vi "PreProcess.vi"(8 "error in (no error)":errorcluster, 11 "Input":T2) -> (0 "error out":errorcluster, 3 "Output":T1)   [LabVIEW 2023]
uses:
  <userlib>/WebService/_PreProcess/PreProcess.lvlib
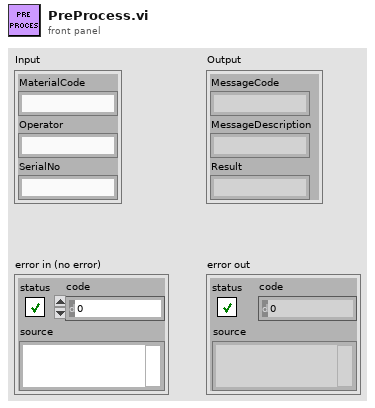
[diagram p1: front panel]
types:
  T1 = cluster{"MessageCode":string, "MessageDescription":string, "Result":string}
  T2 = cluster{"MaterialCode":string, "Operator":string, "SerialNo":string}
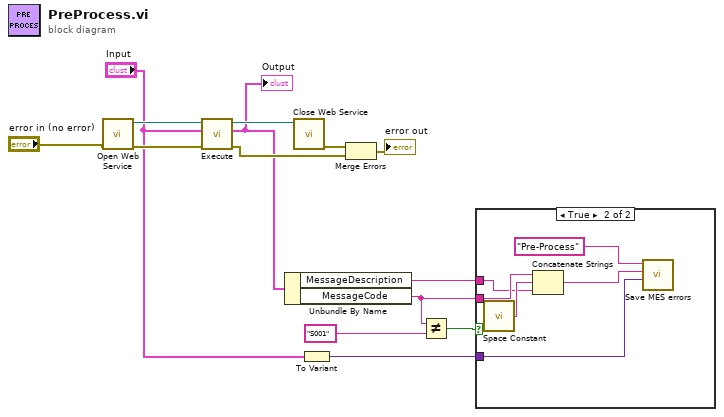
[diagram p0: block diagram]
diagram:
  n1 = call <userlib>:"Open Web Service.vi"("error in (no error)"="error in (no error)") -> ("error out"=w13:errorcluster, "PreProcess refnum"=w14:refnum<k24>)  [unwired: 9 in]
  n2 = call <userlib>:"Execute.vi"("error in (no error)"=w13, ".NET:CheckPqmNtrsAndProductSerialDateService.PqmNtrsAndProductSerialRequest"="Input", "PreProcess refnum"=w14) -> ("error out"=w8:errorcluster, ".NET:CheckPqmNtrsAndProductSerialDateService.CommonResponse"=w2:T1, "PreProcess refnum out"=w12:refnum<k24>)  [unwired: 6 in]
  "Output" <- w2
  n3 = Unbundle By Name(w2) -> ("MessageDescription"=w5:string, "MessageCode"=w4:string)
  n4 = call <userlib>:"Close Web Service.vi"("PreProcess refnum"=w12) -> ("error out"=w10:errorcluster)  [unwired: 10 in]
  n5 = To Variant(anything="Input") -> (Variant=w3:variant)
  n6 = Merge Errors(w10, w8) -> (→"error out":errorcluster)
  n7 = Not Equal?(x=w4, y="S001") -> (x != y?=w7:bool)
  n8 = case shown="True" w7 {
    tunnel: w5 -> [_ w18]
    tunnel: w4 -> [_ w20]
    tunnel: w3 -> [_ w15]
    frame False {
    }
    frame True {
      n9 = call <vilib>:"Space Constant.vi"() -> ("String"=w19:string)
      n10 = Concatenate Strings(w20, w19, w18) -> (w17:string)
      n11 = call "Save MES errors.vi"("Sent parameters"=w15, "Error Text"=w17, "Operation"="Pre-Process") -> ()  [unwired: 9 in]
    }
  }
